vi "Create Data Log.vi"(8 "error in (no error)":errorcluster, 11 "Model in":refnum<class "Model.lvclass">) -> (0 "error out":errorcluster, 3 "Model out":refnum<class "Model.lvclass">)   [LabVIEW 2016, in "Model.lvclass"]
uses:
  Model.lvclass
  Typedefs/TestLogTypes.ctl
  Test Log/Test Log Factory/Test Log Factory.lvclass
  Model.lvclass/Model.ctl
  Test Log/Test Log/Test Log.lvclass
  Typedefs/FAMT Typedefs.lvlib
panel:
  in  "error in (no error) 2":errorcluster
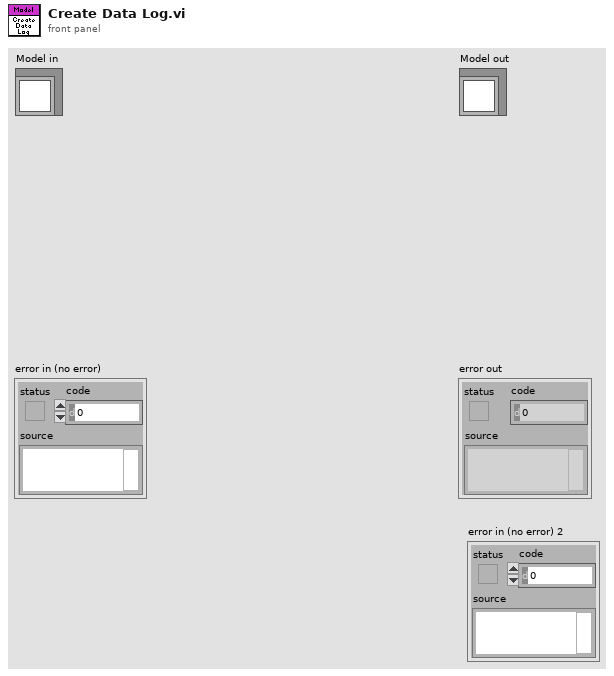
[diagram p1: front panel]
types:
  T1 = typedef "FAMT Typedefs.lvlib/TestLogTypes.ctl" = enum16{"CSV Test Log"}
  T2 = typedef "FAMT Typedefs.lvlib/TestSettings.ctl" = cluster{"Operator":string, "Notes":string, "Actuator Serial Number":string, "Test Stand Serial Number":string, "Axial Load Cell Sensitivity":dbl, "Lateral Load Cell Sensitivity":dbl, "Actuator Type":T3}
  T3 = typedef "RTFAILC.lvlib/FATypes.ctl" = enum16{"SingleAxis", "LateralDualAxis", "CrossLateralDualAxis"}
  T4 = typedef "FAMT Typedefs.lvlib/ActuatorSetPoints.ctl" = cluster{"Axial Force":dbl, "Lateral Force":dbl, "FC1 Force":dbl, "FC2 Force":dbl}
  T5 = typedef "FAMT Typedefs.lvlib/ToveyEngData.ctl" = cluster{"Timestamp":dbl, "Fx":dbl, "Fy":dbl, "Fz":dbl, "Mx":dbl, "My":dbl, "Mz":dbl}
  T6 = typedef "FAMT Typedefs.lvlib/ActuatorData.ctl" = cluster{"Timestamp":dbl, "Axial Force":dbl, "Lateral Force":dbl, "FC1 Force":dbl, "FC2 Force":dbl, "Lateral Push Pressure":dbl, "Lateral Pull Pressure":dbl, "Axial Push Pressure":dbl, "Axial Pull Pressure":dbl}
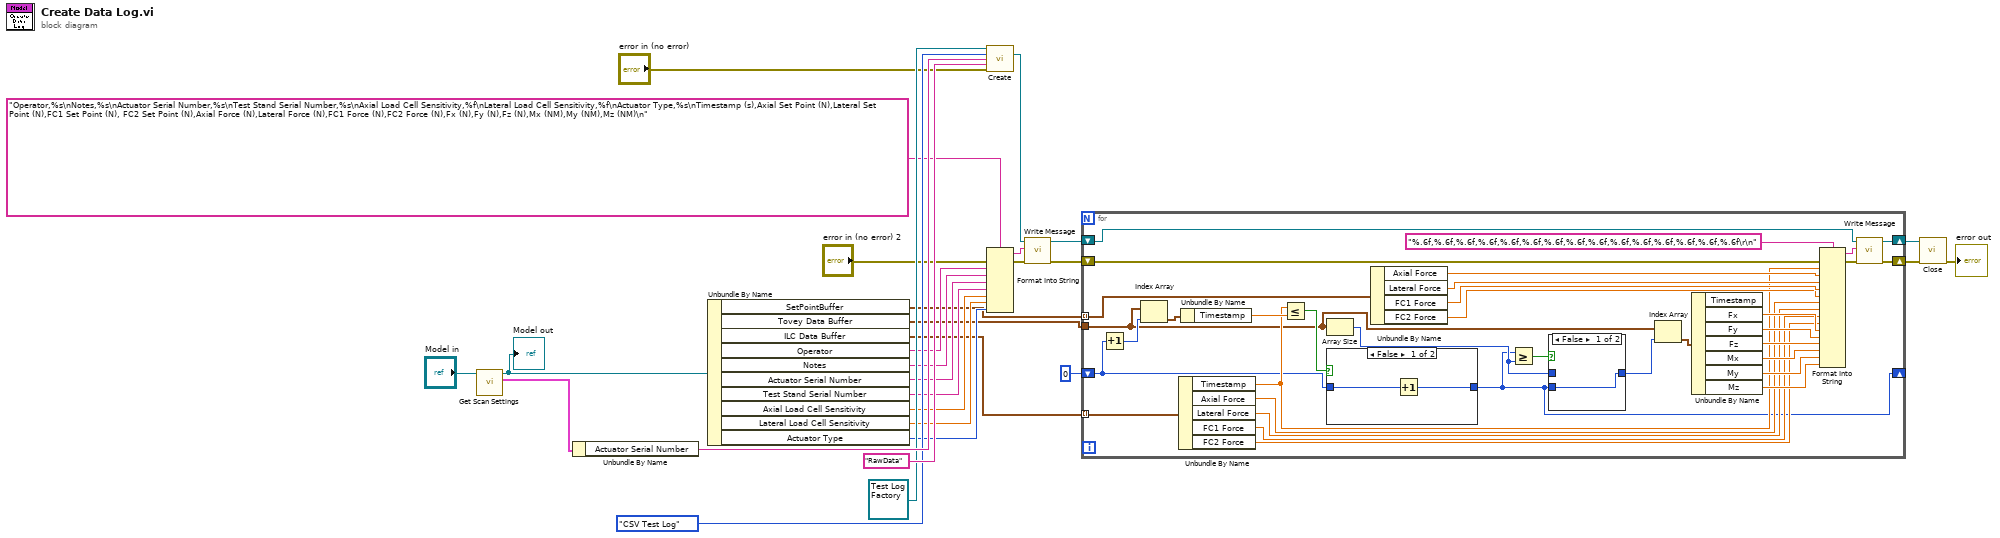
[diagram p0: block diagram]
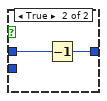
[diagram p2: hidden frame]
diagram:
  n1 = call "Get Scan Settings.vi"("Model in"="Model in") -> ("Test Settings"=w26:T2, "Model out"=w6:refnum<class "Model.lvclass">)  [unwired: 9 in]
  "Model out" <- w6
  n2 = Unbundle By Name(w26) -> ("Actuator Serial Number"=w28:string)
  n3 = Unbundle By Name(w6) -> ("SetPointBuffer"=w9:T4[], "Tovey Data Buffer"=w10:T5[], "ILC Data Buffer"=w2:T6[], "Operator"=w15:string, "Notes"=w17:string, "Actuator Serial Number"=w18:string, "Test Stand Serial Number"=w19:string, "Axial Load Cell Sensitivity"=w20:dbl, "Lateral Load Cell Sensitivity"=w21:dbl, "Actuator Type"=w22:T3)
  n4 = call-dynamic "Create.vi"("Test Log Factory in"=refnum<class "Test Log Factory.lvclass"> refnum ("Test Log Factory.lvclass"), "Test Log Types"=TestLogTypes."CSV Test Log" ("TestLogTypes"), "Test Name"=w28, "Scan Name"="RawData", "error in (no error)"="error in (no error)") -> ("Test Log"=w11:refnum<class "Test Log.lvclass">)  [unwired: 8 in, 2 out]
  n5 = Format Into String(format string="Operator,%s\nNotes,%s\nActuator Serial Number,%s\nTest Stand Serial Number,%s\nAxial Load Cell Sensitivity,%f\nLateral Load Cell Sensitivity,%f\nActuator Type,%s\nTimestamp (s),Axial Set Point (N),Lateral Set Point (N),FC1 Set Point (N), FC2 Set Point (N),Axial Force (N),Lateral Force (N),FC1 Force (N),FC2 Force (N),Fx (N),Fy (N),Fz (N),Mx (NM),My (NM),Mz (NM)\n", error in="error in (no error) 2", w15, w17, w18, w19, w20, w21, w22) -> (resulting string=w12:string, error out=w13:errorcluster)  [unwired: 1 in]
  n6 = call-dynamic "Write Message.vi"("error in (no error)"=w13, "Message"=w12, "Test Log in"=w11) -> ("error out"=w3:errorcluster, "Test Log out"=w4:refnum<class "Test Log.lvclass">)  [unwired: 7 in]
  n7 = for {
    tunnel: w10 -> [w34]
    shift-right: [w62] -> w8
    shift-left: w4 -> [w63]
    shift-right: [w58] -> w7
    shift-left: w3 -> [w61]
    tunnel: w9 -> [w57] mode=indexing
    tunnel: w2 -> [w46] mode=indexing
    shift-right: [w31] -> _
    shift-left: 0 -> [w36]
    n8 = Increment(x=w36) -> (x+1=w35:i32)
    n9 = Index Array(array=w34, index=w35) -> (element=w45:T5)
    n10 = Unbundle By Name(w46) -> ("Timestamp"=w41:dbl, "Axial Force"=w40:dbl, "Lateral Force"=w39:dbl, "FC1 Force"=w38:dbl, "FC2 Force"=w37:dbl)
    n11 = Unbundle By Name(w45) -> ("Timestamp"=w44:dbl)
    n12 = Less Or Equal?(x=w41, y=w44) -> (x <= y?=w43:bool)
    n13 = Array Size(array=w34) -> (size(s)=w32:i32)
    n14 = case shown="False" w43 {
      tunnel: w36 -> [w69 w70]
      tunnel: [w68 w70] -> w31
      frame False {
        n15 = Increment(x=w69) -> (x+1=w68:i32)
      }
      frame True {
      }
    }
    n16 = Unbundle By Name(w57) -> ("Axial Force"=w56:dbl, "Lateral Force"=w55:dbl, "FC1 Force"=w54:dbl, "FC2 Force"=w53:dbl)
    n17 = Greater Or Equal?(x=w31, y=w32) -> (x >= y?=w33:bool)
    n18 = case shown="False" w33 {
      tunnel: w32 -> [_ w67]
      tunnel: [w65 w66] -> w30
      tunnel: w31 -> [w65 _]
      frame False {
      }
      frame True {
        n19 = Decrement(x=w67) -> (x-1=w66:i32)
      }
    }
    n20 = Index Array(array=w34, index=w30) -> (element=w42:T5)
    n21 = Unbundle By Name(w42) -> ("Fx"=w52:dbl, "Fy"=w51:dbl, "Fz"=w50:dbl, "Mx"=w49:dbl, "My"=w48:dbl, "Mz"=w47:dbl)  [unwired: 1 out]
    n22 = Format Into String(format string="%.6f,%.6f,%.6f,%.6f,%.6f,%.6f,%.6f,%.6f,%.6f,%.6f,%.6f,%.6f,%.6f,%.6f,%.6f\r\n", error in=w61, w41, w56, w55, w54, w53, w40, w39, w38, w37, w52, w51, w50, w49, w48, w47) -> (resulting string=w59:string, error out=w60:errorcluster)  [unwired: 1 in]
    n23 = call-dynamic "Write Message.vi"("error in (no error)"=w60, "Message"=w59, "Test Log in"=w63) -> ("error out"=w58:errorcluster, "Test Log out"=w62:refnum<class "Test Log.lvclass">)  [unwired: 7 in]
  }
  n24 = call-dynamic "Close.vi"("error in (no error)"=w7, "Test Log in"=w8) -> ("error out"=→"error out":errorcluster)  [unwired: 8 in, 1 out]
